vi "Read INI Scaling File.vi"(8 "error in":errorcluster, 11 "Path":path) -> (0 "error out":errorcluster, 2 "Scaling Coefficients":T1)   [LabVIEW 2018, in "AE75TX Actor.lvlib" / "AE75TX.lvclass"]
uses:
  AE75TX.lvclass
  Controls/Scaling Coefficients Measurements.ctl
  <vilib>/Utility/config.llb/NI_LVConfig.lvlib
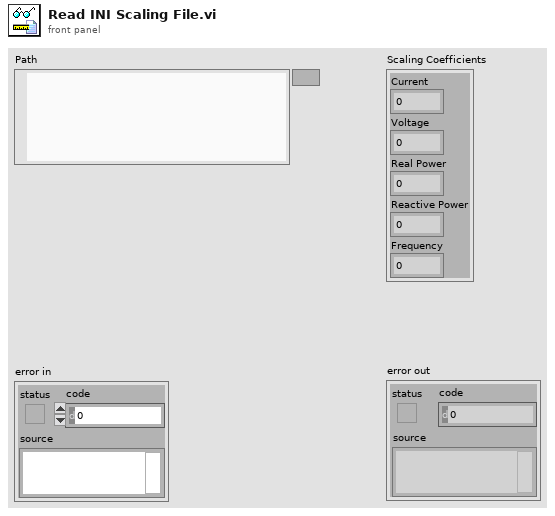
[diagram p1: front panel]
types:
  T1 = typedef "AE75TX Actor.lvlib/AE75TX.lvclass/Scaling Coefficients Measurements.ctl" = cluster{"Current":dbl, "Voltage":dbl, "Real Power":dbl, "Reactive Power":dbl, "Frequency":dbl}
  T2 = typedef "NI_LVConfig.lvlib/Config Data RefNum.ctl" = refnum<k1>
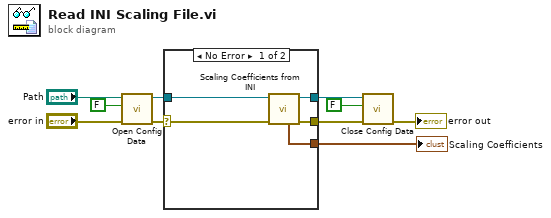
[diagram p0: block diagram]
diagram:
  n1 = call <vilib>:"Open Config Data.vi"("error in (no error)"="error in", "create file if necessary (T)"=FALSE, "configuration file path"="Path") -> ("error out"=w8:errorcluster, "refnum"=w7:T2)  [unwired: 6 in, 1 out]
  n2 = case shown="No Error" w8 {
    selector: w8 -> [w12 w16]
    tunnel: w7 -> [w13 w17]
    tunnel: [w15 w17] -> w6
    tunnel: [w14 w16] -> w5
    tunnel: [w11 _] -> w1
    frame No Error {
      n3 = call "Scaling Coefficients from INI.vi"("error in"=w12, "Config Refnum in"=w13) -> ("error out"=w14:errorcluster, "Config Refnum out"=w15:T2, "Scaling Coefficients"=w11:T1)  [unwired: 7 in]
    }
    frame Error {
    }
  }
  "Scaling Coefficients" <- w1
  n4 = call <vilib>:"Close Config Data.vi"("error in (no error)"=w5, "write file if changed (T)"=FALSE, "refnum"=w6) -> ("error out"=→"error out":errorcluster)  [unwired: 7 in, 1 out]
